vi "main_fg.vi"() -> ()   [LabVIEW 2015]
uses:
  <vilib>/Instr/_visa.llb/VISA Configure Serial Port (Instr).vi
panel:
  out "Reading":bool
  out "Writing":bool
  out "Numeric 2":i32
  out "Numeric":i32
  out "initialized array":string[](array[string])
  out "VISA resource name out 2":refnum<visa-resource-name>
  out "error out 2":errorcluster
  in  "error get_value":errorcluster
  in  "Get status":bool
  in  "Attenuation":string(combo)
  in  "Level":dbl
  in  "Cmos":string(combo)
  in  "Duty":dbl
  in  "Modulation":string(combo)
  in  "Frequency":dbl=0.0001 min=0.0 max=0.5 step=0.001
  in  "Range":string(combo)
  in  "Offset":dbl
  in  "Counter":string(combo)
  out "error out":errorcluster
  in  "Function type":string(combo)
  in  "close":bool=TRUE
  out "VISA resource name out":refnum<visa-resource-name>
  in  "open":bool=TRUE
  in  "VISA resource name":refnum<visa-resource-name>
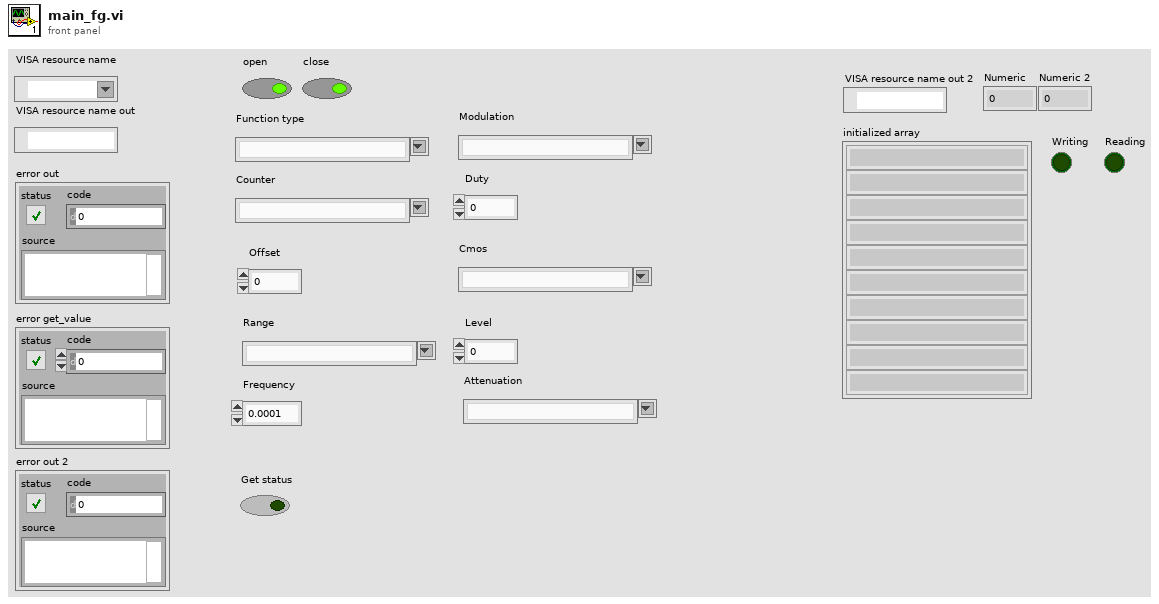
[diagram p1: front panel]
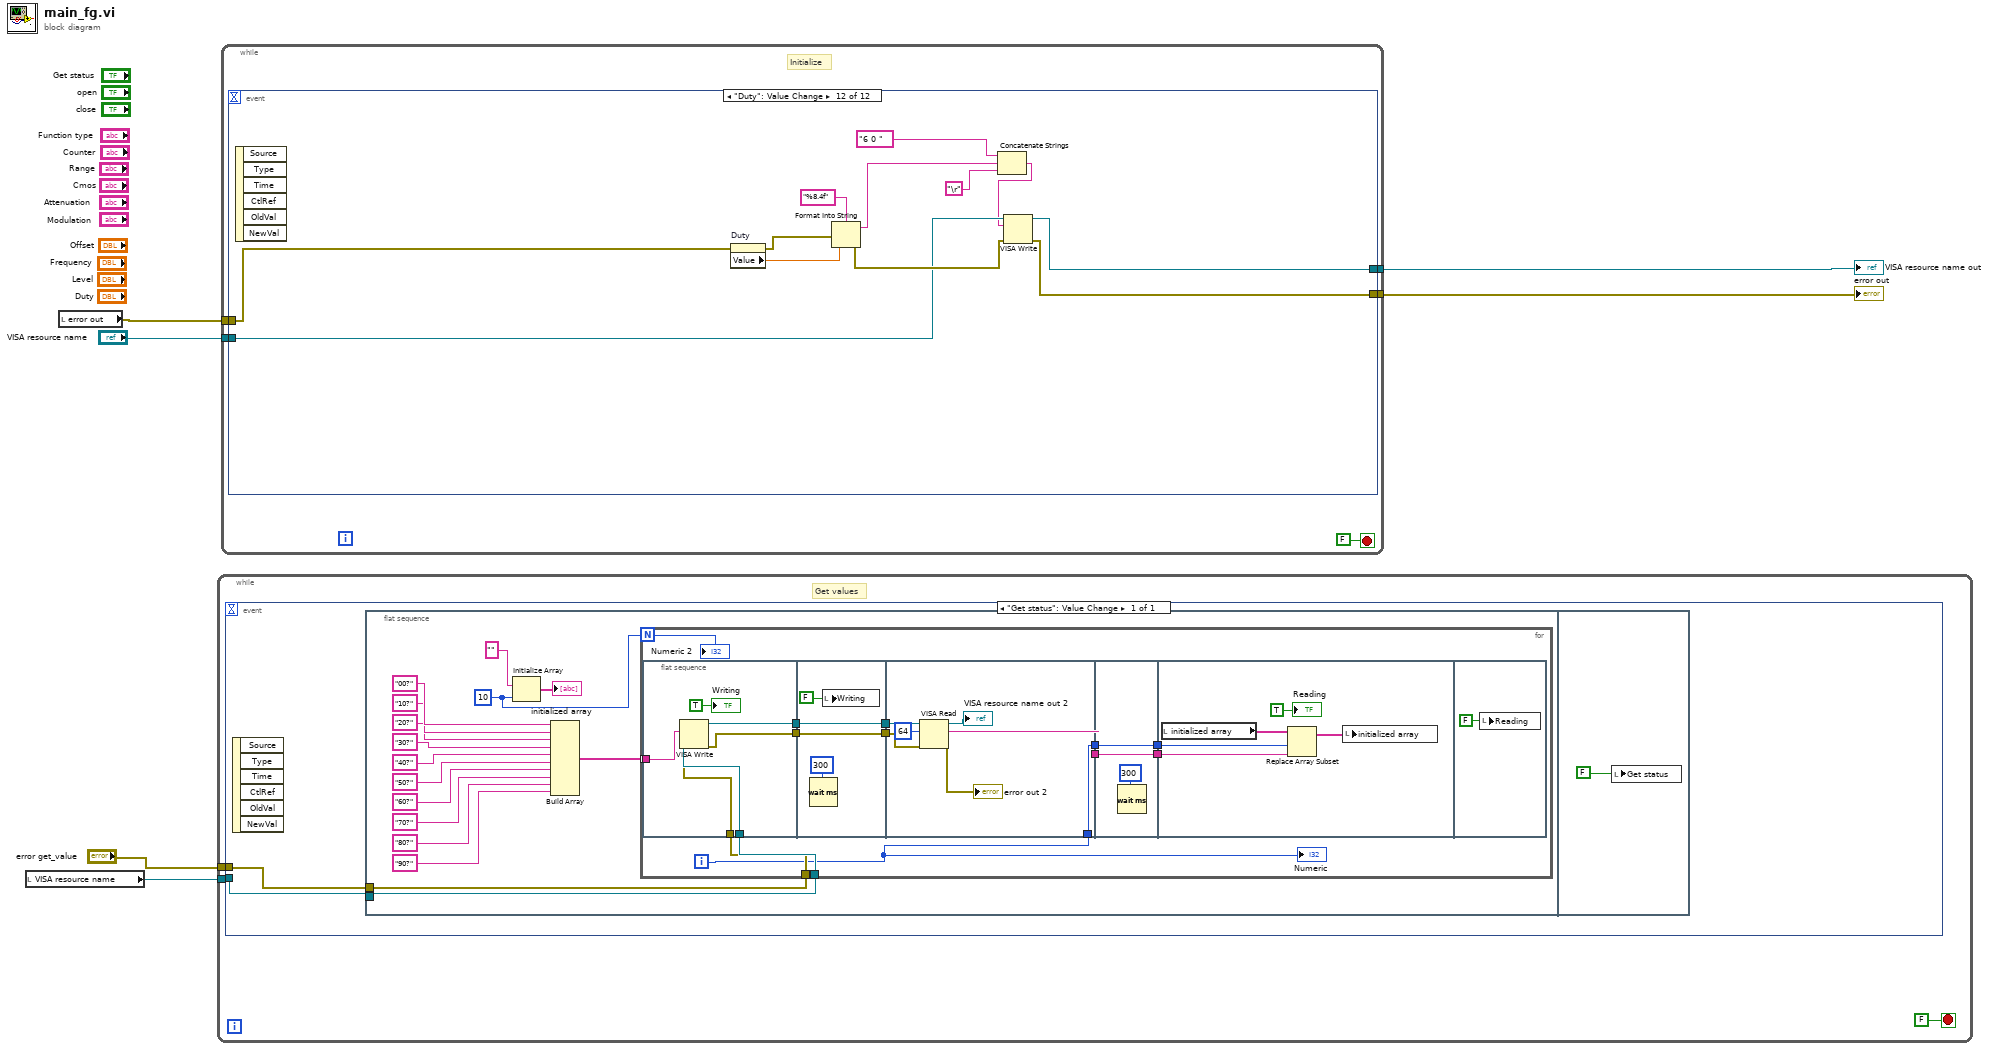
[diagram p0: block diagram]
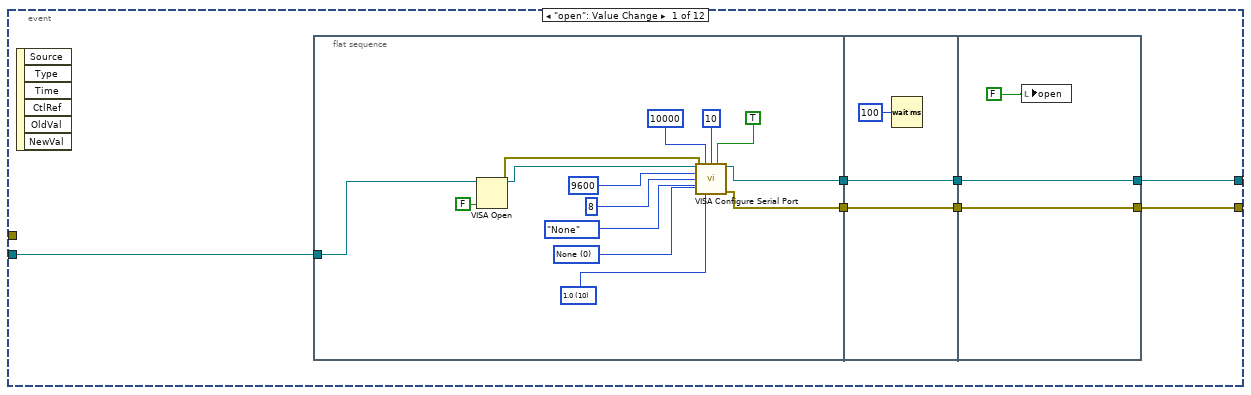
[diagram p2: hidden frame]
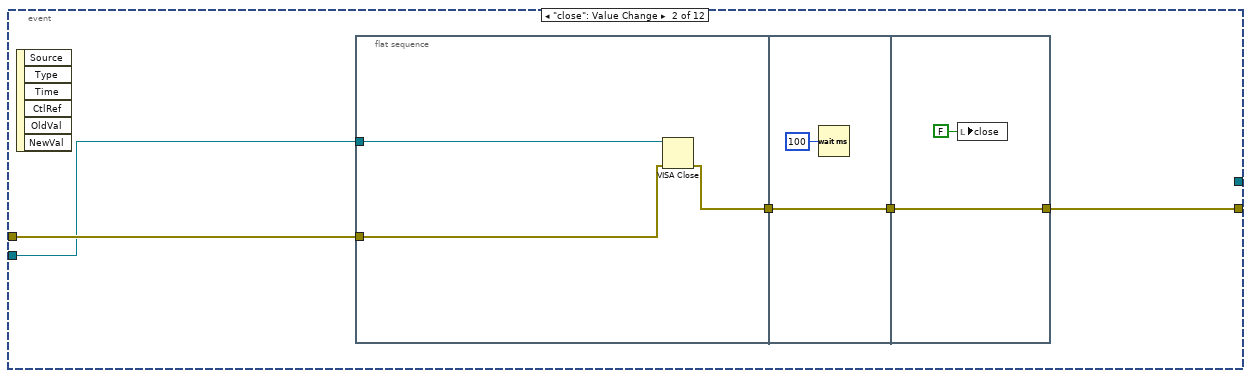
[diagram p3: hidden frame]
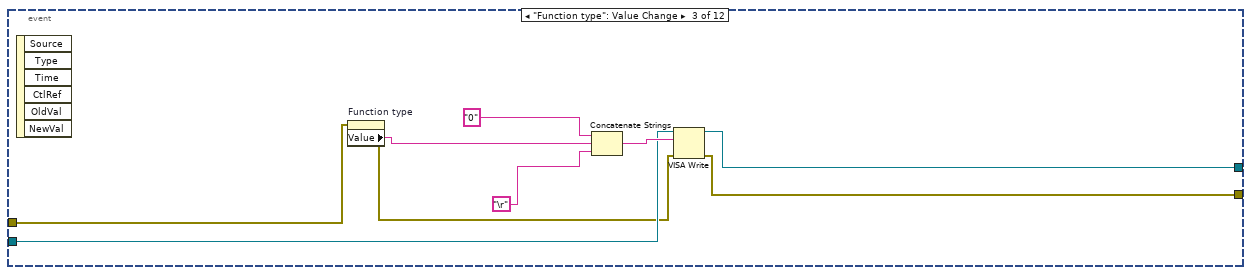
[diagram p4: hidden frame]
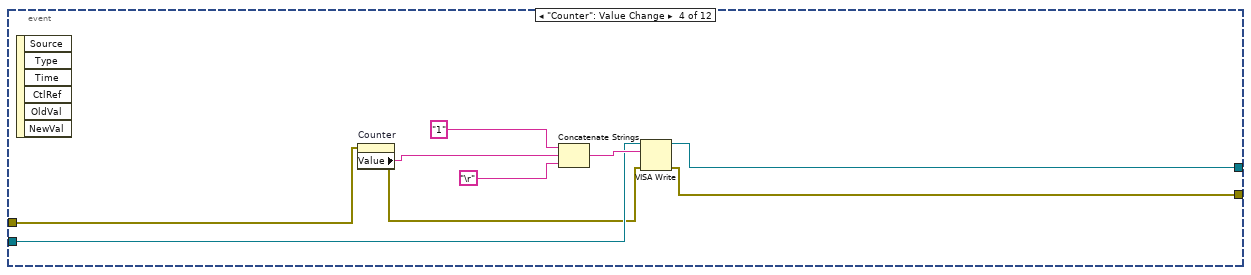
[diagram p5: hidden frame]
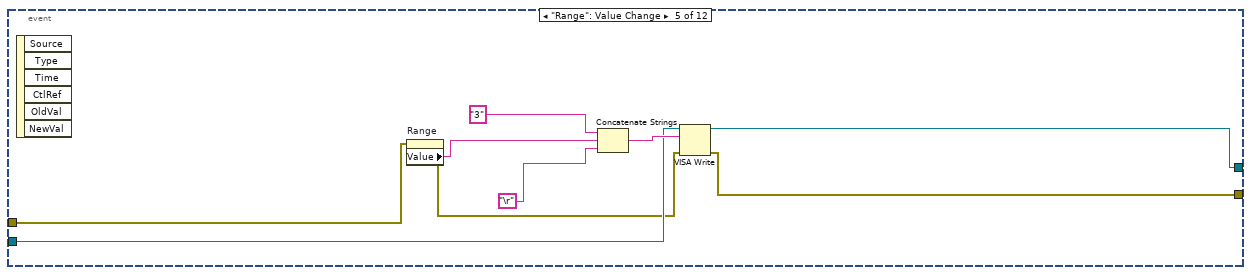
[diagram p6: hidden frame]
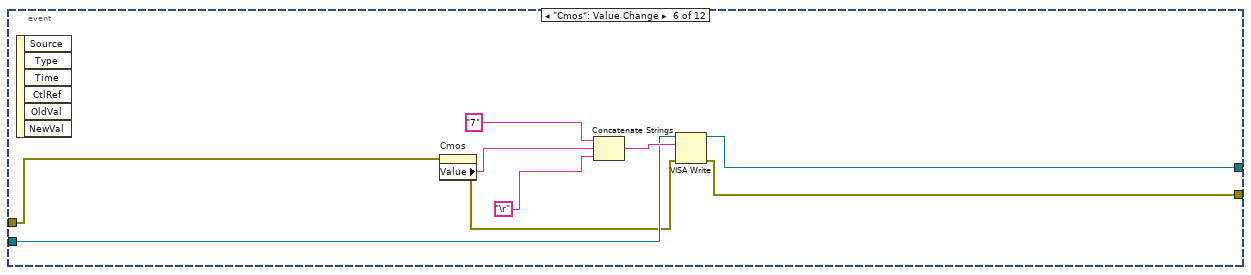
[diagram p7: hidden frame]
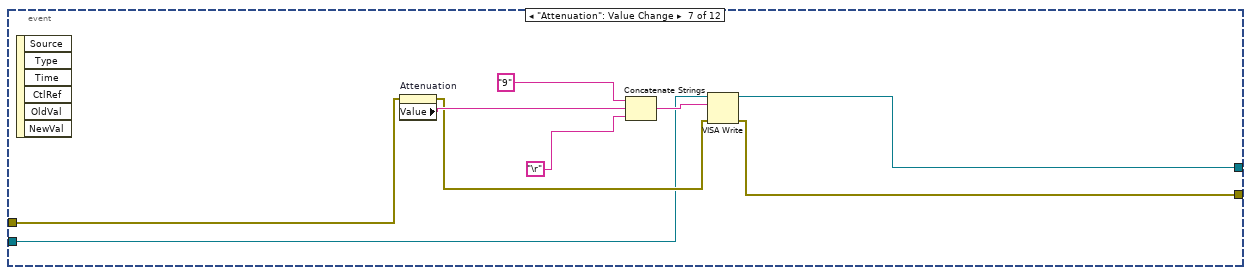
[diagram p8: hidden frame]
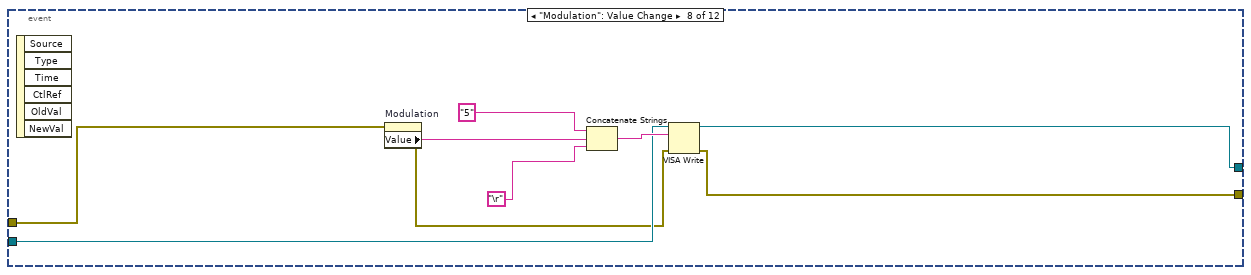
[diagram p9: hidden frame]
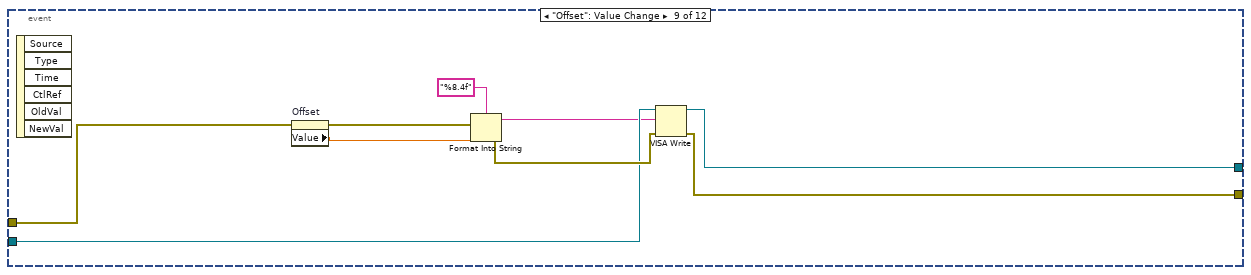
[diagram p10: hidden frame]
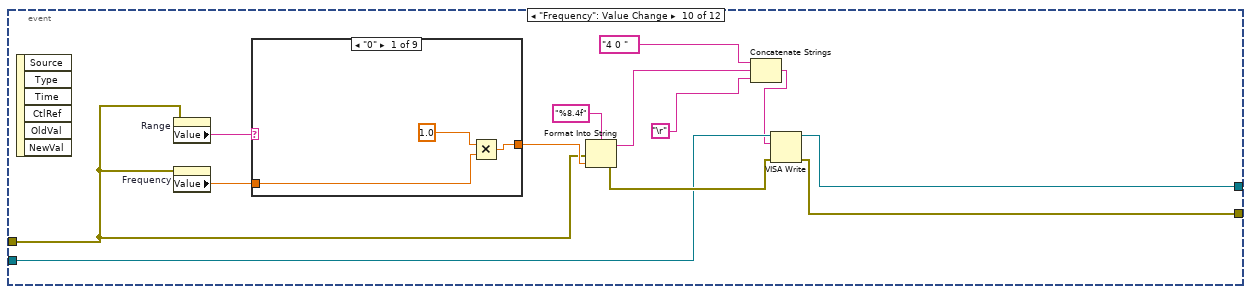
[diagram p11: hidden frame]
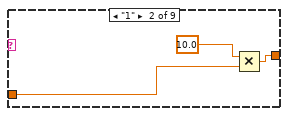
[diagram p12: hidden frame]
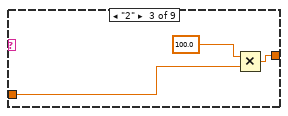
[diagram p13: hidden frame]
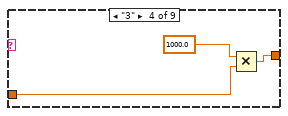
[diagram p14: hidden frame]
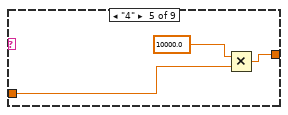
[diagram p15: hidden frame]
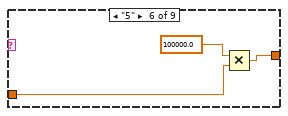
[diagram p16: hidden frame]
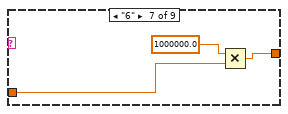
[diagram p17: hidden frame]
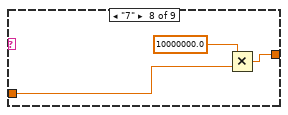
[diagram p18: hidden frame]
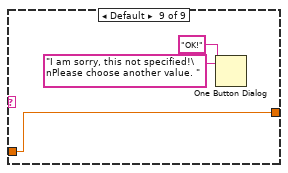
[diagram p19: hidden frame]
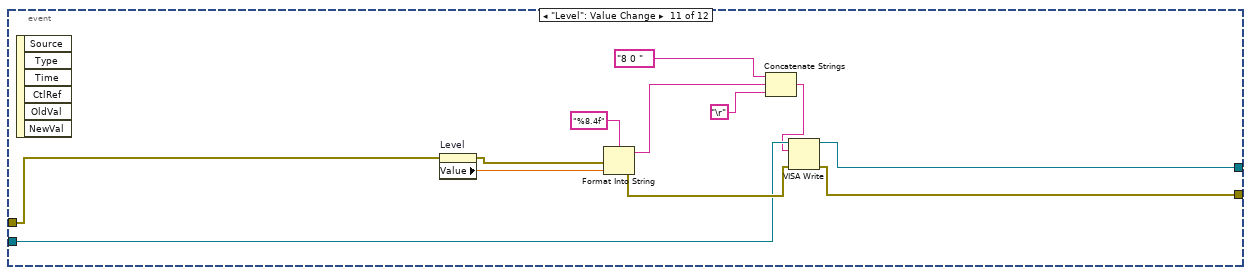
[diagram p20: hidden frame]
diagram:
  n1 = local read "VISA resource name"() -> (w2:refnum<visa-resource-name>)
  n2 = local read "error out"() -> (w6:errorcluster)
  n3 = while {
    tunnel: w2 -> [w8]
    tunnel: "error get_value" -> [w7]
    stop <- FALSE stop-if-true
    # "Get values"
    n4 = event shown="[0] \"Get status\": Value Change" {
      selector: _ -> [_]
      dyn-events: _ -> [_]
      timeout: _ -> [_]
      tunnel: w8 -> [w11]
      tunnel: w7 -> [w10]
      event "Get status": Value Change {
        n5 = event-data() -> ()  [unwired: 1 in, 6 out]
        n6 = flat-sequence {
          tunnel: w11 -> [w16]
          tunnel: w10 -> [w15]
          frame #0 {
            w12 = 10 ("dimension size")
            n7 = Initialize Array("", w12) -> (→"initialized array":string[])
            n8 = Build Array("00?", "10?", "20?", "30?", "40?", "50?", "60?", "70?", "80?", "90?") -> (w17:string[])
            n9 = for {
              N: w12 -> [w28]
              tunnel: w17 -> [w38] mode=indexing
              tunnel: w16 -> [w40]
              tunnel: w15 -> [w39]
              i -> [w37]
              n10 = flat-sequence {
                tunnel: w40 -> [w46]
                tunnel: [w45] -> w36
                tunnel: [w44] -> w34
                tunnel: w39 -> [w43]
                tunnel: w38 -> [w42]
                tunnel: w36 -> [w50]
                tunnel: [w50] -> w35
                tunnel: w34 -> [w49]
                tunnel: [w49] -> w33
                tunnel: w35 -> [w57]
                tunnel: w33 -> [w56]
                tunnel: w37 -> [w52]
                tunnel: [w52] -> w32
                tunnel: [w51] -> w30
                tunnel: w32 -> [w60]
                tunnel: [w60] -> w31
                tunnel: w30 -> [w59]
                tunnel: [w59] -> w29
                tunnel: w31 -> [w63]
                tunnel: w29 -> [w64]
                frame #0 {
                  n11 = VISA Write(VISA resource name=w46, write buffer=w42, error in (no error)=w43) -> (VISA resource name out=w45:refnum<visa-resource-name>, error out=w44:errorcluster)  [unwired: 1 out]
                  "Writing" <- TRUE ("Reading")
                }
                frame #1 {
                  n12 = Wait (ms)(milliseconds to wait=u32 300) -> ()  [unwired: 1 out]
                  n13 = local write "Writing"(FALSE ("Reading")) -> ()
                }
                frame #2 {
                  n14 = VISA Read(VISA resource name=w57, byte count=u32 64, error in (no error)=w56) -> (VISA resource name out=→"VISA resource name out 2":refnum<visa-resource-name>, read buffer=w51:string, error out=→"error out 2":errorcluster)  [unwired: 1 out]
                }
                frame #3 {
                  n15 = Wait (ms)(milliseconds to wait=u32 300) -> ()  [unwired: 1 out]
                }
                frame #4 {
                  n16 = local read "initialized array"() -> (w65:string[])
                  n17 = Replace Array Subset(array=w65, new element=w64, index=w63) -> (w62:string[])
                  n18 = local write "initialized array"(w62) -> ()
                  "Reading" <- TRUE ("Writing")
                }
                frame #5 {
                  n19 = local write "Reading"(FALSE ("Writing")) -> ()
                }
              }
              "Numeric" <- w37
              "Numeric 2" <- w28
            }
          }
          frame #1 {
            n20 = local write "Get status"(FALSE ("Get status")) -> ()
          }
        }
      }
    }
  }
  n21 = while {
    tunnel: w6 -> [w71]
    tunnel: [w70] -> w5
    tunnel: "VISA resource name" -> [w68]
    tunnel: [w69] -> w3
    stop <- FALSE ("stop") stop-if-true
    # "Initialize"
    n22 = event shown="[11] \"Duty\": Value Change" {
      selector: _ -> [_ _ _ _ _ _ _ _ _ _ _ _]
      dyn-events: _ -> [_ _ _ _ _ _ _ _ _ _ _ _]
      timeout: _ -> [_ _ _ _ _ _ _ _ _ _ _ _]
      tunnel: w71 -> [_ w104 w113 w122 w131 w140 w149 w158 w167 w179 w220 w232]
      tunnel: [w77 w103 w117 w126 w133 w143 w153 w160 w172 w183 w223 w234] -> w70
      tunnel: [w78 _ w115 w125 w134 w142 w152 w161 w169 w184 w222 w235] -> w69
      tunnel: w68 -> [w79 w102 w116 w124 w135 w144 w148 w162 w171 w185 w224 w236]
      event "open": Value Change {
        n23 = event-data() -> ()  [unwired: 1 in, 6 out]
        n24 = flat-sequence {
          tunnel: w79 -> [w92]
          tunnel: [w90] -> w76
          tunnel: [w89] -> w75
          tunnel: w76 -> [w96]
          tunnel: w75 -> [w95]
          tunnel: [w96] -> w74
          tunnel: [w95] -> w73
          tunnel: [w98] -> w77
          tunnel: [w99] -> w78
          tunnel: w74 -> [w99]
          tunnel: w73 -> [w98]
          frame #0 {
            w80 = u16 0 items=["None", "XON/XOFF", "RTS/CTS", "XON/XOFF & RTS/CTS", "DTR/DSR", "XON/XOFF & DTR/DSR"] ("flow control (0:none)")
            w81 = u16 10 items=["1.0"=10, "1.5"=15, "2.0"=20] ("stop bits (10: 1 bit)")
            n25 = VISA Open(duplicate session (F)=FALSE, VISA resource name=w92) -> (VISA resource name=w91:refnum<visa-resource-name>, error out=w88:errorcluster)  [unwired: 3 in]
            n26 = call-poly "VISA Configure Serial Port"("VISA resource name"=w91, "timeout (10sec)"=u32 10000, "termination char\n(0xA = '\\n' = LF)"=u8 10 ("termination char\n(0xA = '\\n' = LF)"), "Enable Termination\nChar (T)"=TRUE ("Enable Termination\nChar (T)"), "baud rate (9600)"=u32 9600, "data bits (8)"=u16 8, "parity (0:none)"=enum16{"None", "Odd", "Even", "Mark", "Space"}."None", "error in (no error)"=w88, "stop bits (10: 1 bit)"=w81, "flow control (0:none)"=w80) -> ("VISA resource name out"=w90:refnum<visa-resource-name>, "error out"=w89:errorcluster)  [unwired: 4 in]
          }
          frame #1 {
            n27 = Wait (ms)(milliseconds to wait=u32 100) -> ()  [unwired: 1 out]
          }
          frame #2 {
            n28 = local write "open"(FALSE) -> ()
          }
        }
      }
      event "close": Value Change {
        n29 = event-data() -> ()  [unwired: 1 in, 6 out]
        n30 = flat-sequence {
          tunnel: w104 -> [w107]
          tunnel: w102 -> [w105]
          tunnel: [w106] -> w101
          tunnel: w101 -> [w109]
          tunnel: [w109] -> w100
          tunnel: [w111] -> w103
          tunnel: w100 -> [w111]
          frame #0 {
            n31 = VISA Close(VISA resource name=w105, error in (no error)=w107) -> (error out=w106:errorcluster)
          }
          frame #1 {
            n32 = Wait (ms)(milliseconds to wait=u32 100) -> ()  [unwired: 1 out]
          }
          frame #2 {
            n33 = local write "close"(FALSE ("close")) -> ()
          }
        }
      }
      event "Function type": Value Change {
        n34 = event-data() -> ()  [unwired: 1 in, 6 out]
        n35 = property on="Function type" class="CmbBox"(error in=w113) -> (error out=w112:errorcluster, "Value"=w114:string)  [unwired: 1 in, 1 out]
        n36 = Concatenate Strings("0" ("string"), w114, "\r") -> (w119:string)
        n37 = VISA Write(VISA resource name=w116, write buffer=w119, error in (no error)=w112) -> (VISA resource name out=w115:refnum<visa-resource-name>, error out=w117:errorcluster)  [unwired: 1 out]
      }
      event "Counter": Value Change {
        n38 = event-data() -> ()  [unwired: 1 in, 6 out]
        n39 = property on="Counter" class="CmbBox"(error in=w122) -> (error out=w121:errorcluster, "Value"=w123:string)  [unwired: 1 in, 1 out]
        n40 = Concatenate Strings("1" ("string"), w123, "\r") -> (w128:string)
        n41 = VISA Write(VISA resource name=w124, write buffer=w128, error in (no error)=w121) -> (VISA resource name out=w125:refnum<visa-resource-name>, error out=w126:errorcluster)  [unwired: 1 out]
      }
      event "Range": Value Change {
        n42 = event-data() -> ()  [unwired: 1 in, 6 out]
        n43 = property on="Range" class="CmbBox"(error in=w131) -> (error out=w130:errorcluster, "Value"=w132:string)  [unwired: 1 in, 1 out]
        n44 = Concatenate Strings("3" ("string"), w132, "\r") -> (w137:string)
        n45 = VISA Write(VISA resource name=w135, write buffer=w137, error in (no error)=w130) -> (VISA resource name out=w134:refnum<visa-resource-name>, error out=w133:errorcluster)  [unwired: 1 out]
      }
      event "Cmos": Value Change {
        n46 = event-data() -> ()  [unwired: 1 in, 6 out]
        n47 = property on="Cmos" class="CmbBox"(error in=w140) -> (error out=w139:errorcluster, "Value"=w141:string)  [unwired: 1 in, 1 out]
        n48 = Concatenate Strings("7" ("string"), w141, "\r") -> (w146:string)
        n49 = VISA Write(VISA resource name=w144, write buffer=w146, error in (no error)=w139) -> (VISA resource name out=w142:refnum<visa-resource-name>, error out=w143:errorcluster)  [unwired: 1 out]
      }
      event "Attenuation": Value Change {
        n50 = event-data() -> ()  [unwired: 1 in, 6 out]
        n51 = property on="Attenuation" class="CmbBox"(error in=w149) -> (error out=w150:errorcluster, "Value"=w151:string)  [unwired: 1 in, 1 out]
        n52 = Concatenate Strings("9" ("string"), w151, "\r") -> (w155:string)
        n53 = VISA Write(VISA resource name=w148, write buffer=w155, error in (no error)=w150) -> (VISA resource name out=w152:refnum<visa-resource-name>, error out=w153:errorcluster)  [unwired: 1 out]
      }
      event "Modulation": Value Change {
        n54 = event-data() -> ()  [unwired: 1 in, 6 out]
        n55 = property on="Modulation" class="CmbBox"(error in=w158) -> (error out=w157:errorcluster, "Value"=w159:string)  [unwired: 1 in, 1 out]
        n56 = Concatenate Strings("5" ("string"), w159, "\r") -> (w164:string)
        n57 = VISA Write(VISA resource name=w162, write buffer=w164, error in (no error)=w157) -> (VISA resource name out=w161:refnum<visa-resource-name>, error out=w160:errorcluster)  [unwired: 1 out]
      }
      event "Offset": Value Change {
        n58 = event-data() -> ()  [unwired: 1 in, 6 out]
        n59 = property on="Offset" class="DigNum (strict)"(error in=w167) -> (error out=w166:errorcluster, "Value"=w168:dbl)  [unwired: 1 in, 1 out]
        n60 = Format Into String(format string="%8.4f", error in=w166, w168) -> (resulting string=w170:string, error out=w173:errorcluster)  [unwired: 1 in]
        n61 = VISA Write(VISA resource name=w171, write buffer=w170, error in (no error)=w173) -> (VISA resource name out=w169:refnum<visa-resource-name>, error out=w172:errorcluster)  [unwired: 1 out]
      }
      event "Frequency": Value Change {
        n62 = event-data() -> ()  [unwired: 1 in, 6 out]
        n63 = property on="Range" class="CmbBox"(error in=w179) -> ("Value"=w180:string)  [unwired: 1 in, 2 out]
        n64 = property on="Frequency" class="DigNum (strict)"(error in=w179) -> ("Value"=w181:dbl)  [unwired: 1 in, 2 out]
        n65 = case shown="\"0\"" w180 {
          tunnel: w181 -> [w189 w192 w195 w198 w201 w204 w207 w210 w214]
          tunnel: [w188 w191 w194 w197 w200 w203 w206 w209 w214] -> w182
          frame "0" {
            n66 = Multiply(x=1.0 ("Frequency"), y=w189) -> (x*y=w188:dbl)
          }
          frame "1" {
            n67 = Multiply(x=10.0 ("Frequency"), y=w192) -> (x*y=w191:dbl)
          }
          frame "2" {
            n68 = Multiply(x=100.0 ("Frequency"), y=w195) -> (x*y=w194:dbl)
          }
          frame "3" {
            n69 = Multiply(x=1000.0 ("Frequency"), y=w198) -> (x*y=w197:dbl)
          }
          frame "4" {
            n70 = Multiply(x=10000.0 ("Frequency"), y=w201) -> (x*y=w200:dbl)
          }
          frame "5" {
            n71 = Multiply(x=100000.0 ("Frequency"), y=w204) -> (x*y=w203:dbl)
          }
          frame "6" {
            n72 = Multiply(x=1000000.0 ("Frequency"), y=w207) -> (x*y=w206:dbl)
          }
          frame "7" {
            n73 = Multiply(x=10000000.0 ("Frequency"), y=w210) -> (x*y=w209:dbl)
          }
          frame Default {
            n74 = One Button Dialog(message="I am sorry, this not specified!\nPlease choose another value. ", button name ("OK")="OK!") -> ()  [unwired: 1 out]
          }
        }
        n75 = Format Into String(format string="%8.4f", error in=w179, w182) -> (resulting string=w176:string, error out=w186:errorcluster)  [unwired: 1 in]
        n76 = Concatenate Strings("4 0 " ("string"), w176, "\r") -> (w175:string)
        n77 = VISA Write(VISA resource name=w185, write buffer=w175, error in (no error)=w186) -> (VISA resource name out=w184:refnum<visa-resource-name>, error out=w183:errorcluster)  [unwired: 1 out]
      }
      event "Level": Value Change {
        n78 = event-data() -> ()  [unwired: 1 in, 6 out]
        n79 = property on="Level" class="DigNum (strict)"(error in=w220) -> (error out=w219:errorcluster, "Value"=w221:dbl)  [unwired: 1 in, 1 out]
        n80 = Format Into String(format string="%8.4f", error in=w219, w221) -> (resulting string=w216:string, error out=w225:errorcluster)  [unwired: 1 in]
        n81 = Concatenate Strings("8 0 " ("string"), w216, "\r") -> (w217:string)
        n82 = VISA Write(VISA resource name=w224, write buffer=w217, error in (no error)=w225) -> (VISA resource name out=w222:refnum<visa-resource-name>, error out=w223:errorcluster)  [unwired: 1 out]
      }
      event "Duty": Value Change {
        n83 = event-data() -> ()  [unwired: 1 in, 6 out]
        n84 = property on="Duty" class="DigNum (strict)"(error in=w232) -> (error out=w231:errorcluster, "Value"=w233:dbl)  [unwired: 1 in, 1 out]
        n85 = Format Into String(format string="%8.4f", error in=w231, w233) -> (resulting string=w228:string, error out=w237:errorcluster)  [unwired: 1 in]
        n86 = Concatenate Strings("6 0 " ("string"), w228, "\r") -> (w227:string)
        n87 = VISA Write(VISA resource name=w236, write buffer=w227, error in (no error)=w237) -> (VISA resource name out=w235:refnum<visa-resource-name>, error out=w234:errorcluster)  [unwired: 1 out]
      }
    }
  }
  "error out" <- w5
  "VISA resource name out" <- w3
